vi "FR XCL Write measurement line.vi"(6 "Iteration index":i32, 7 "report in":refnum<class "NI_report.lvclass">, 8 "error in (no error)":errorcluster, 9 "TWM result as string for XCL":string[][](array[string]), 10 "DC readings":dbl[](array[numeric]), 11 "FR measurement":T1={"Measurement frequencies (Hz)"=[1000.0, 10000.0, 1000.0], "Sampling frequency (Hz)"=500000.0, "Signal amplitude (V)"=4.5, "AC-DC settle time (s)"=20.0, "Record length (multiples of period)"=[1000.0, 10000.0, 1000.0], "Measurement template file"=path "", "Row of START keyword"=0, "Row of STOP keyword"=0, "Calculate RMS from samples"=FALSE, "AC-DC warm up time (s)"=300.0, "Measurement template line"=[], "DC meter readings No."=10, "Algorithm"="TWM-WFFT", "Simultaneous measurement"=FALSE, "Recalculate-skip already calculated"=FALSE} {"Record length (multiples of period)" format="%#_3p"; "Sampling frequency (Hz)" format="%#_3p"; "Measurement frequencies (Hz)" format="%#_3p"}) -> (0 "error out":errorcluster, 5 "report out":refnum<class "NI_report.lvclass">)   [LabVIEW 2020]
doc: "Writes measurement results for a single line in FR template."
uses:
  <vilib>/Utility/NIReport.llb/NI_report.lvclass
  FR Measurement/Type definitions/FR measuement.ctl
  external libraries/varilib/varilib.lvlib
  <vilib>/Analysis/NI_AALBase.lvlib
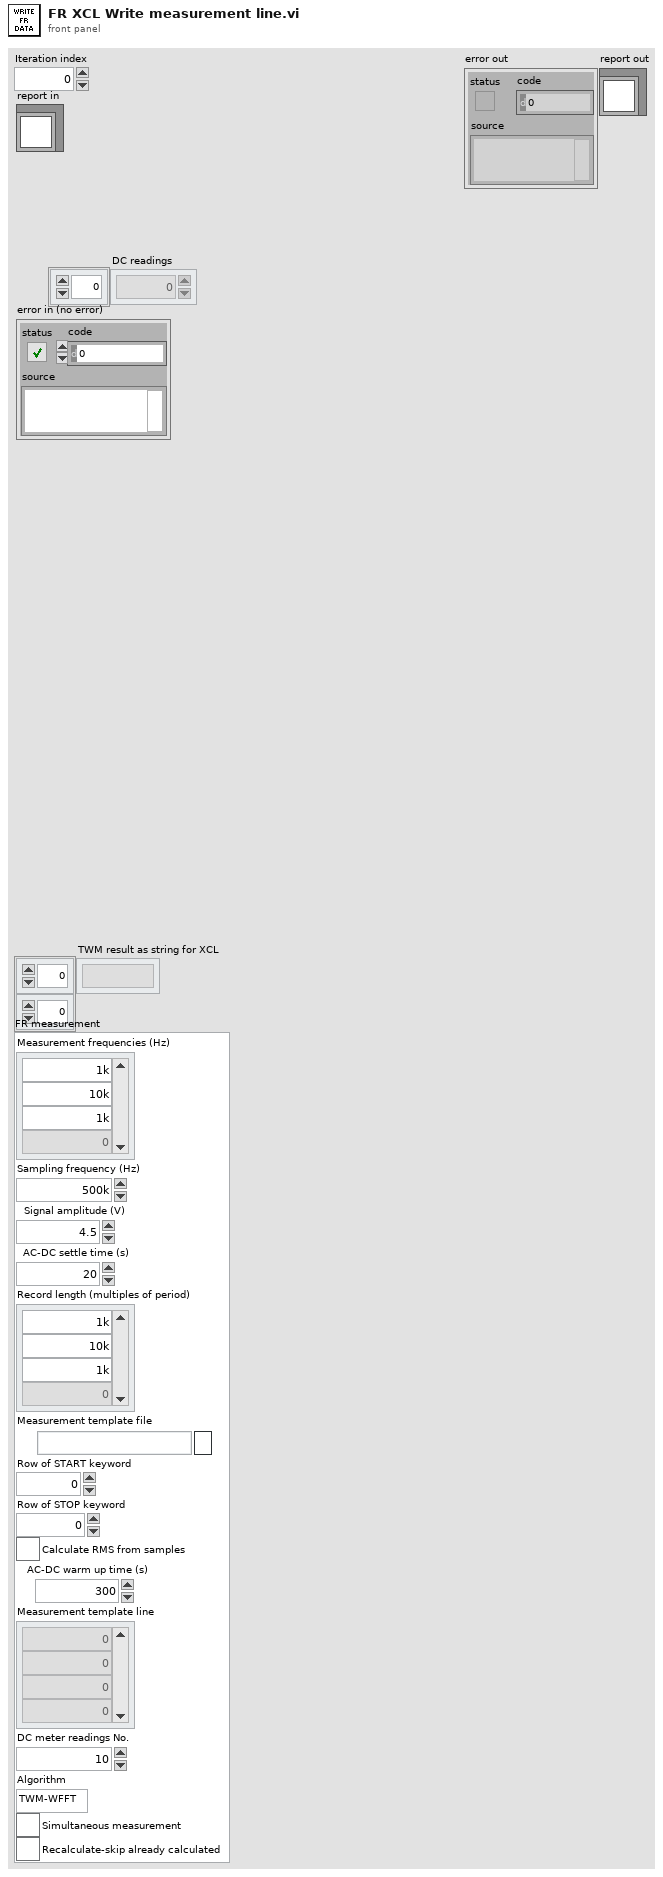
[diagram p1: front panel]
types:
  T1 = typedef "FR measuement.ctl" = cluster{"Measurement frequencies (Hz)":dbl[], "Sampling frequency (Hz)":dbl, "Signal amplitude (V)":dbl, "AC-DC settle time (s)":dbl, "Record length (multiples of period)":dbl[], "Measurement template file":path, "Row of START keyword":i32, "Row of STOP keyword":i32, "Calculate RMS from samples":bool, "AC-DC warm up time (s)":dbl, "Measurement template line":i32[], "DC meter readings No.":i32, "Algorithm":string, "Simultaneous measurement":bool, "Recalculate-skip already calculated":bool}
  T2 = typedef "Type definitions to be saved.ctl" = cluster{"Common properties":T3, "AC Source":T4, "DC meter":T6, "CE measurement":T8, "FR measurement":T1, "FR template":T9, "CE template":T10, "PJVS":T11, "SS measurement":T15, "AC sync source":T4}
  T3 = typedef "Common properties.ctl" = cluster{"Measurement status ref":refnum<vi>, "TWM Status ref":refnum<vi>, "Abort ref":refnum<vi>, "Skip waiting ref":refnum<vi>, "GNU Octave path":path, "TWM+QWTB path":path, "lvlib path":path, "TWM pipe":string, "PJVS status ref":refnum<vi>, "WAC path":path}
  T4 = typedef "AC Source.ctl" = cluster{"AC Source type":T5, "VISA":refnum<visa-resource-name>, "Ref. clock (Hz)":dbl, "status ref":refnum<vi>, "Fluke 57XX wideband output":bool, "Fluke 57XX ignore errors":bool, "Synchronization by AC signal":bool}
  T5 = typedef "AC Source type.ctl" = enum16{"Fluke 5XXX calibrator", "Tektronix AFG3000 series", "dummy", "Agilent 331xxA to 332xxA", "Agilent 335xxA to 336xxA"}
  T6 = typedef "DC meter.ctl" = cluster{"DC meter type":T7, "DC meter VISA":refnum<visa-resource-name>, "NPLC":dbl, "status ref":refnum<vi>}
  T7 = typedef "DC meter type.ctl" = enum16{"H/A/K 3458", "Fluke 8508A", "dummy", "Keithley 2182"}
  T8 = typedef "CE measurement.ctl" = cluster{"Signal frequencies (Hz) T":dbl[], "Signal amplitudes (V) T":dbl[], "Sampling frequencies (Hz) T":dbl[], "Record lengths (multiples of periods) T":dbl[], "TWM data root directory":path, "TWM mreasurements directories":path[], "Calculate RMS from samples":bool, "RMS algorithm T":string, "Settle down after AC source change (s) T":dbl, "Skip PJVS setup":bool, "Measurement template file":path, "Row of START keyword T":i32, "Row of STOP keyword T":i32, "Measurement template line T":i32[], "Switch position T":dbl[], "FR fit mat file T":path, "Recalculate-skip already calculated":bool}
  T9 = typedef "FR template.ctl" = cluster{"Keywords column":i32, "Sig. freq. column":i32, "Rec. len. column":i32, "Meas. points. row min to read":i32, "Meas. points. row max to read":i32, "Properties column":i32, "Properties row start":i32, "Properties row end":i32, "Keyword START regexp":string, "Keyword STOP regexp":string, "HW data column":i32, "HW data row start":i32, "HW data row end":i32, "TIme and date column start":i32, "Digitizer value column start ":i32, "DC mean column start ":i32, "DC readings column start":i32}
  T10 = typedef "CE template.ctl" = cluster{"Keywords column":i32, "Sig. freq. column":i32, "Rec. len. column":i32, "Switch pos column":i32, "Meas. points. row min to read":i32, "Meas. points. row max to read":i32, "Properties column":i32, "Properties row start":i32, "Properties row end":i32, "Keyword START regexp":string, "Keyword STOP regexp":string, "HW data column":i32, "HW data row start":i32, "HW data row end":i32, "TIme and date column start":i32, "Digitizer value column start ":i32}
  T11 = typedef "PJVS.ctl" = cluster{"PJVS type":T12, "Status Refnum":refnum<vi>, "AC-supraVOLTcontrol":cluster{"IP address:port (0.0.0.0:0000)":string, "Timeouts":T13, "Simulation mode":bool, "Debug mode":bool}, "NPL bias source":cluster{"DataSocketCluster":T14}, "Manual PJVS":cluster{"PJVS frequency (Hz)":dbl, "Reference voltages (V)":dbl[], "File with PJVS voltages":path}, "VTT PJVS":cluster{"some VTT only property":string}}
  T12 = typedef "PJVS Type.ctl" = enum16{"AC-supraVOLTcontrol", "JV modified NPL bias control", "Manual PJVS", "VTT PJVS"}
  T13 = typedef "ACSVcontrol-driver.lvlib/Timeouts.ctl" = cluster{"TCP Read & Write (ms)":i32, "Sensors readout":i32, "PJVS setup":i32, "Nullmeter readout":i32, "Multiplexer setup":i32, "57XX setup":i32, "Generator setup":i32, "Synthesizer setup":i32, "Sampler readout":i32}
  T14 = typedef "DataSocketCluster external.ctl" = cluster{"Server Machine":string, "Client Machine":string, "Data":string, "TimeStamp":dbl, "Count":i32, "Target Process":string}
  T15 = typedef "SS measurement.ctl" = cluster{"Signal frequencies (Hz)":dbl[], "Signal amplitudes (V)":dbl[], "Sampling frequencies (Hz)":dbl[], "Record lengths (multiples of periods)":dbl[], "Calculate results":bool, "Algorithm":string, "TWM data directories":path[], "TWM data directories relative":path[], "Settle down after AC source change (s)":dbl, "PJVS frequencies (Hz)":dbl[], "PJVS reference voltages array of vector cluster":cluster{"PJVS reference voltages vector":dbl[]}[], "Requested PJVS steps":u32[], "Measure CE":bool, "Measure CE before":bool, "Measure CE after":bool, "Single point CE measurement":bool, "original CE template path":path, "new CE template path before SS":path, "new CE template path before SS relative":path, "new CE template path after SS":path, "new CE template path after SS relative":path, "original CE fit path":path, "new CE fit path before SS":path, "new CE fit path before SS relative":path, "new CE fit path after SS":path, "new CE fit path after SS relative":path, "Measure digitizer gain":bool, "Measure digitizer gain before":bool, "Measure digitizer gain after":bool, "Digitizer gain":dbl, "Data folder":path, "FR fit path":path, "new FR fit path relative":path, "Rs":i32, "Re":i32, "SS measurement info files":path[]}
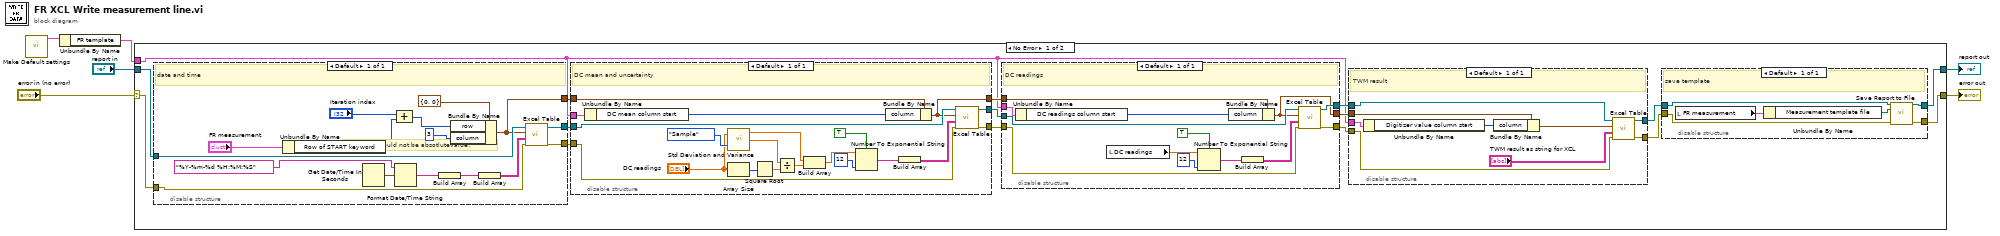
[diagram p0: block diagram]
diagram:
  n1 = call "Make Default settings.vi"() -> ("TD to be saved"=w2:T2)  [unwired: 11 in]
  n2 = Unbundle By Name(w2) -> ("FR template"=w1:T9)
  n3 = case shown="No Error" "error in (no error)" {
    selector: "error in (no error)" -> [w22 w88]
    tunnel: [w20 w88] -> w6
    tunnel: "report in" -> [w21 w87]
    tunnel: [w19 w87] -> w3
    tunnel: w1 -> [w7 _]
    frame No Error {
      n4 = disable-structure shown="Default" {
        disable-tunnel: w22 -> [w80]
        disable-tunnel: w21 -> [w79]
        disable-tunnel: [w78] -> w18
        disable-tunnel: [w77] -> w17
        disable-tunnel: [w76] -> w16
        frame Enabled {
          # "#XXX this should not be absotlutevalue!"
          # "date and time"
          n5 = Unbundle By Name("FR measurement") -> ("Row of START keyword"=w72:i32)
          n6 = Get Date/Time In Seconds() -> (seconds since 1Jan1904=w82:timestamp)
          n7 = Format Date/Time String(time format string (%c)="%Y-%m-%d %H:%M:%S", seconds (now)=w82) -> (date/time string=w84:string)  [unwired: 1 in]
          n8 = Compound Arithmetic op=ADD("Iteration index", w72) -> (w75:i32)
          n9 = Build Array(w84) -> (w85:string[])
          n10 = Bundle By Name(cluster=cluster{"row":i32, "column":i32} {"row"=0, "column"=0} ("start (0, 0)"), "row"=w75, "column"=3) -> (w76:cluster{"row":i32, "column":i32})
          n11 = Build Array(w85) -> (w86:string[][])
          n12 = call "Excel Table.vi"("error in (no error)"=w80, "table"=w86, "start (0, 0)"=w76, "report in"=w79) -> ("error out"=w78:errorcluster, "report out"=w77:refnum<class "NI_report.lvclass">)  [unwired: 6 in]
        }
      }
      n13 = disable-structure shown="Default" {
        disable-tunnel: w18 -> [w68]
        disable-tunnel: w17 -> [w67]
        disable-tunnel: w16 -> [w64]
        disable-tunnel: [w63] -> w11
        disable-tunnel: [w62] -> w13
        disable-tunnel: [w61] -> w12
        disable-tunnel: w7 -> [w52]
        frame Enabled {
          # "DC mean and uncertainty"
          n14 = Unbundle By Name(w52) -> ("DC mean column start"=w51:i32)
          n15 = call <vilib>:"Std Deviation and Variance.vi"("X"="DC readings", "Weighting (Sample)"=enum16{"Sample", "Population"}."Sample") -> ("mean"=w57:dbl, "standard deviation"=w58:dbl)  [unwired: 1 out]
          n16 = Array Size(array="DC readings") -> (size(s)=w54:i32)
          n17 = Square Root(x=w54) -> (sqrt(x)=w59:dbl)
          n18 = Divide(x=w58, y=w59) -> (x/y=w56:dbl)
          n19 = Build Array(w57, w56) -> (w55:dbl[])
          n20 = Number To Exponential String(number=w55, precision (6)=i16 12, 1:TRUE ("use system decimal point (T)")) -> (E-format string=w66:string[])  [unwired: 1 in]
          n21 = Bundle By Name(cluster=w64, "column"=w51) -> (w61:cluster{"row":i32, "column":i32})
          n22 = Build Array(w66) -> (w65:string[][])
          n23 = call "Excel Table.vi"("error in (no error)"=w68, "table"=w65, "start (0, 0)"=w61, "report in"=w67) -> ("error out"=w63:errorcluster, "report out"=w62:refnum<class "NI_report.lvclass">)  [unwired: 6 in]
        }
      }
      n24 = disable-structure shown="Default" {
        disable-tunnel: w11 -> [w39]
        disable-tunnel: w13 -> [w38]
        disable-tunnel: w12 -> [w35]
        disable-tunnel: [w34] -> w10
        disable-tunnel: [w33] -> w8
        disable-tunnel: [w32] -> w9
        disable-tunnel: w7 -> [w30]
        frame Enabled {
          # "DC readings"
          n25 = Unbundle By Name(w30) -> ("DC readings column start"=w29:i32)
          n26 = local read "DC readings"() -> (w31:dbl[])
          n27 = Number To Exponential String(number=w31, precision (6)=i16 12, 1:TRUE ("use system decimal point (T)")) -> (E-format string=w37:string[])  [unwired: 1 in]
          n28 = Bundle By Name(cluster=w35, "column"=w29) -> (w32:cluster{"row":i32, "column":i32})
          n29 = Build Array(w37) -> (w36:string[][])
          n30 = call "Excel Table.vi"("error in (no error)"=w39, "table"=w36, "start (0, 0)"=w32, "report in"=w38) -> ("error out"=w34:errorcluster, "report out"=w33:refnum<class "NI_report.lvclass">)  [unwired: 6 in]
        }
      }
      n31 = disable-structure shown="Default" {
        disable-tunnel: w10 -> [w50]
        disable-tunnel: w8 -> [w49]
        disable-tunnel: [w48] -> w15
        disable-tunnel: [w47] -> w14
        disable-tunnel: w9 -> [w46]
        disable-tunnel: w7 -> [w43]
        frame Enabled {
          # "TWM result"
          n32 = Unbundle By Name(w43) -> ("Digitizer value column start"=w42:i32)
          n33 = Bundle By Name(cluster=w46, "column"=w42) -> (w45:cluster{"row":i32, "column":i32})
          n34 = call "Excel Table.vi"("error in (no error)"=w50, "table"="TWM result as string for XCL", "start (0, 0)"=w45, "report in"=w49) -> ("error out"=w48:errorcluster, "report out"=w47:refnum<class "NI_report.lvclass">)  [unwired: 6 in]
        }
      }
      n35 = disable-structure shown="Default" {
        disable-tunnel: [w28] -> w20
        disable-tunnel: [w27] -> w19
        disable-tunnel: w15 -> [w26]
        disable-tunnel: w14 -> [w25]
        frame Enabled {
          # "save template"
          n36 = local read "FR measurement"() -> (w24:T1)
          n37 = Unbundle By Name(w24) -> ("Measurement template file"=w23:path)
          n38 = call-dynamic "Save Report to File.vi"("report in"=w25, "report file path"=w23, "error in (no error)"=w26) -> ("report out"=w27:refnum<class "NI_report.lvclass">, "error out"=w28:errorcluster)  [unwired: 11 in]
        }
      }
    }
    frame Error {
    }
  }
  "error out" <- w6
  "report out" <- w3
